vi "FMPA Wait for Process Complete.vi"(8 "error in":errorcluster, 10 "Routines to query":string[](array[string]), 11 "System no.":i32) -> (0 "error out":errorcluster, 3 "Status":i32[](array[numeric]))   [LabVIEW 2023]
panel:
  out "XY Graph":cluster{dbl[], dbl[]}(graph)
  in  "Polling time in ms":u32=1
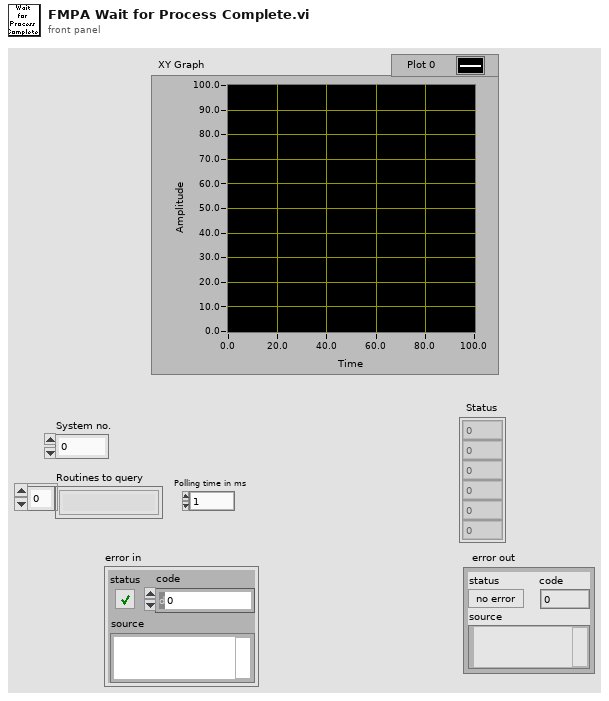
[diagram p1: front panel]
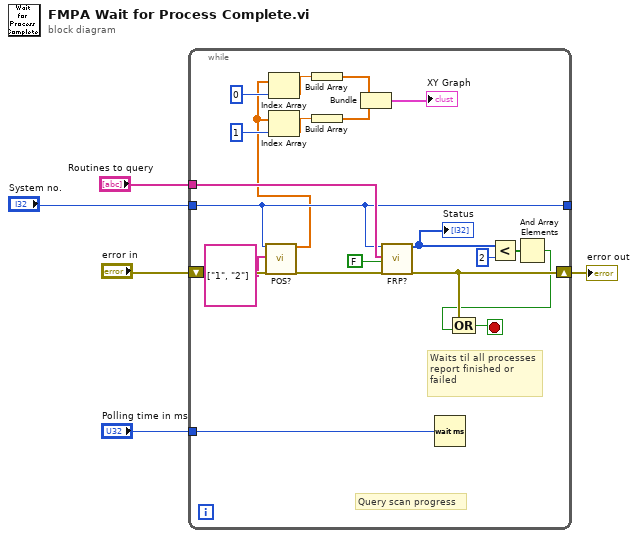
[diagram p0: block diagram]
diagram:
  n1 = while {
    shift-right: [w22] -> w1
    shift-left: "error in" -> [w17]
    tunnel: "System no." -> [w15]
    tunnel: "Routines to query" -> [w18]
    tunnel: "Polling time in ms" -> [w21]
    tunnel: [w15] -> _
    stop <- w26 stop-if-true
    # "Waits til all processes\nreport finished or\nfailed"
    # "Query scan progress"
    n2 = call "POS?.vi"("System no."=w15, "Axes to query"=string[] ["1", "2"], "error in"=w17) -> ("Position"=w11:dbl[], "error out"=w16:errorcluster)  [unwired: 15 in]
    n3 = Index Array(array=w11, index=0) -> (element=w10:dbl)
    n4 = Index Array(array=w11, index=1) -> (element=w9:dbl)
    n5 = Build Array(w10) -> (w8:dbl[])
    n6 = Build Array(w9) -> (w7:dbl[])
    n7 = Bundle(w8, w7) -> (→"XY Graph":cluster{dbl[], dbl[]})  [unwired: 1 in]
    n8 = call "FRP?.vi"("System no."=w15, "Routines to query"=w18, "All routines?"=FALSE, "error in"=w16) -> ("Status"=w20:i32[], "error out"=w22:errorcluster)  [unwired: 14 out]
    "Status" <- w20
    n9 = Wait (ms)(milliseconds to wait=w21) -> ()  [unwired: 1 out]
    n10 = Less?(x=w20, y=2) -> (x < y?=w23:bool[])
    n11 = And Array Elements(Boolean array=w23) -> (logical AND=w19:bool)
    n12 = Compound Arithmetic op=OR(w22, w19) -> (w26:bool)
  }
  "error out" <- w1
